vi "Gateway_Initialise.vi"(8 "error in (no error)":errorcluster, 11 "GatewayClass in":refnum<class "GatewayClass.lvclass">) -> (0 "error out":errorcluster, 3 "GatewayClass out":refnum<class "GatewayClass.lvclass">)   [LabVIEW 2018, in "feGEM Gateway.lvlib" / "GatewayClass.lvclass"]
uses:
  GatewayClass.lvclass
  DataPacker/DataStructures/GEM_BANK_ARRAY.lvclass
  DataPacker/DataStructures/GEM_BANK_CLUSTER_typedef.ctl
  DataPacker/DataStructures/GEM_DATA_cluster_typedef.ctl
  GatewayClass.lvclass/GatewayClass.ctl
  4c942e19-3362-4030-94fa-f0a52f440fa1.vi
  feGEM DataPacker.lvlib
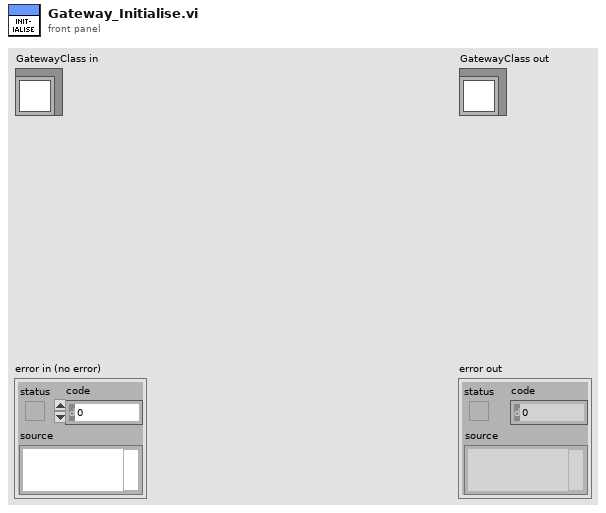
[diagram p1: front panel]
types:
  T1 = enum16{"big-endian, network order", "native, host order", "little-endian"}
  T2 = typedef "feGEM DataPacker.lvlib/GEM_BANK_CLUSTER_typedef.ctl" = cluster{"Category":string, "Variable Name":string, "Equipment description":string, "History Settings":u16, "Period to update history plots":u16, "GEM_DATA Cluster":T3}
  T3 = typedef "feGEM DataPacker.lvlib/GEM_DATA_cluster_typedef.ctl" = cluster{"DataType":string, "Formatted Data":u8[], "data byte order (Little Endian prefered)":enum16{"big-endian, network order", "native, host order", "little-endian"}}
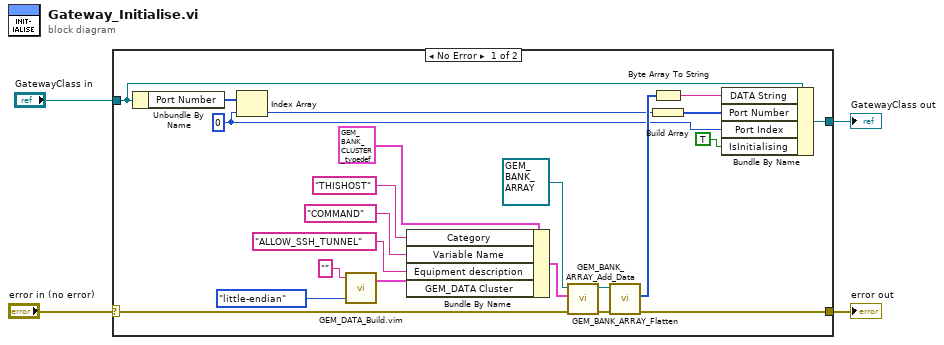
[diagram p0: block diagram]
diagram:
  n1 = case shown="No Error" "error in (no error)" {
    selector: "error in (no error)" -> [w16 w28]
    tunnel: [w15 w28] -> w3
    tunnel: [w13 w27] -> w1
    tunnel: "GatewayClass in" -> [w12 w27]
    frame No Error {
      w8 = 0 ("index")
      n2 = Unbundle By Name(w12) -> ("Port Number"=w11:u16[])
      n3 = Index Array(array=w11, index=w8) -> (element=w10:u16)
      n4 = call "GEM_DATA_Build.vim"("byte order (Little Endian prefered)"=T1."little-endian", "Any array in"="") -> ("GEM_BANK Cluster"=w17:T3)  [unwired: 1 in, 1 out]
      n5 = Bundle By Name(cluster=T2 {"Category"="", "Variable Name"="", "Equipment description"="", "History Settings"=0, "Period to update history plots"=0, "GEM_DATA Cluster"={"DataType"="", "Formatted Data"=[], "data byte order (Little Endian prefered)"=enum."big-endian, network order"}} ("output cluster"), "Category"="THISHOST", "Variable Name"="COMMAND", "Equipment description"="ALLOW_SSH_TUNNEL" ("Variable Name"), "GEM_DATA Cluster"=w17) -> (w25:T2)
      n6 = call "GEM_BANK_ARRAY_Add_Data.vi"("error in (no error)"=w16, "GEM BANK Cluster"=w25, "LVBANKARRAY in"=refnum<class "GEM_BANK_ARRAY.lvclass"> refnum) -> ("error out"=w22:errorcluster, "LVBANKARRAY out"=w23:refnum<class "GEM_BANK_ARRAY.lvclass">)  [unwired: 7 in]
      n7 = call "GEM_BANK_ARRAY_Flatten.vi"("error in (no error)"=w22, "LVBANKARRAY in"=w23) -> ("error out"=w15:errorcluster, "Array"=w21:u8[])  [unwired: 7 in, 1 out]
      n8 = Byte Array To String(unsigned byte array=w21) -> (string=w14:string)
      n9 = Build Array(w10) -> (w9:u16[])
      n10 = Bundle By Name(cluster=w12, "DATA String"=w14, "Port Number"=w9, "Port Index"=w8, "IsInitialising"=TRUE) -> (w13:refnum<class "GatewayClass.lvclass">)
    }
    frame Error {
    }
  }
  "error out" <- w3
  "GatewayClass out" <- w1
